vi "MultiplexerSerialInterfaceQueue.vi"() -> ()   [LabVIEW 2016]
uses:
  controls/Enum.ctl
  <vilib>/rvi/errors/niLvFpgaAdjustHostInterfaceError.vi
  <vilib>/regexp/Match Regular Expression.xnode
  <vilib>/rvi/interface/nirviReadWriteControl/nirviReadWriteControl.xnode
  controls/FPGAVIreferenceTypeDef.ctl
  FPGA Bitfiles/qnmController797_usbRIO_controllerFPGAmu.lvbitx
  Course Project/support/Message Queue/Message Queue.lvlib
  NiFpgaLv.dll
panel:
  in  "Clock delay":u32=1
  in  "QuadMultiplier":T1={"Update Multiplexer"=FALSE, "Adress (0-3)"=1, "Resistance"=0} {"Resistance" max=256; "Adress (0-3)" max=32}
  in  "Buffer":T2={"Update Multiplexer"=FALSE, "CH(0-3)"=1, "Output Voltage"=0.0} {"CH(0-3)" max=4}
  in  "VGA":cluster{"Update":bool, "Gain (0-40) (dB)":u32}={"Update"=FALSE, "Gain (0-40) (dB)"=6} {"Gain (0-40) (dB)" max=40}
  in  "Multiplexer":T3={"Update Multiplexer"=FALSE, "Channel #"=2} {"Channel #" max=32}
  in  "Output Enable":bool
  # "Buffer"
  # "VGA"
  # "HMC960LP4E"
  # "DAC8554"
  # "Quad Multiplier"
  # "Multiplexer"
  # "HV5122"
  # "AD5144"
  # "Update the multiplexer"
  # "Offset"
  # "Filter"
  # "Range"
  # "MICROCHIP"
  # "TEXAS INSTRUMENTS"
  # "Serial to Parallel Converter"
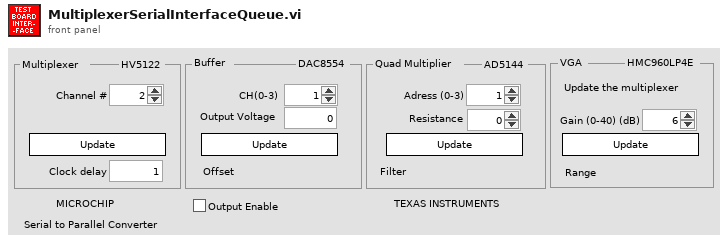
[diagram p1: front panel]
types:
  T1 = cluster{"Update Multiplexer":bool, "Adress (0-3)":u8, "Resistance":u16}
  T2 = cluster{"Update Multiplexer":bool, "CH(0-3)":u8, "Output Voltage":dbl}
  T3 = cluster{"Update Multiplexer":bool, "Channel #":u8}
  T4 = typedef "Message Queue.lvlib/All Message Queues.ctl" = cluster{"IU":refnum<queue>}
  T5 = typedef "Enum.ctl" = enum16{"Init", "Read", "Write"}
  T6 = typedef "FPGAVIreferenceTypeDef.ctl" = refnum<k20>
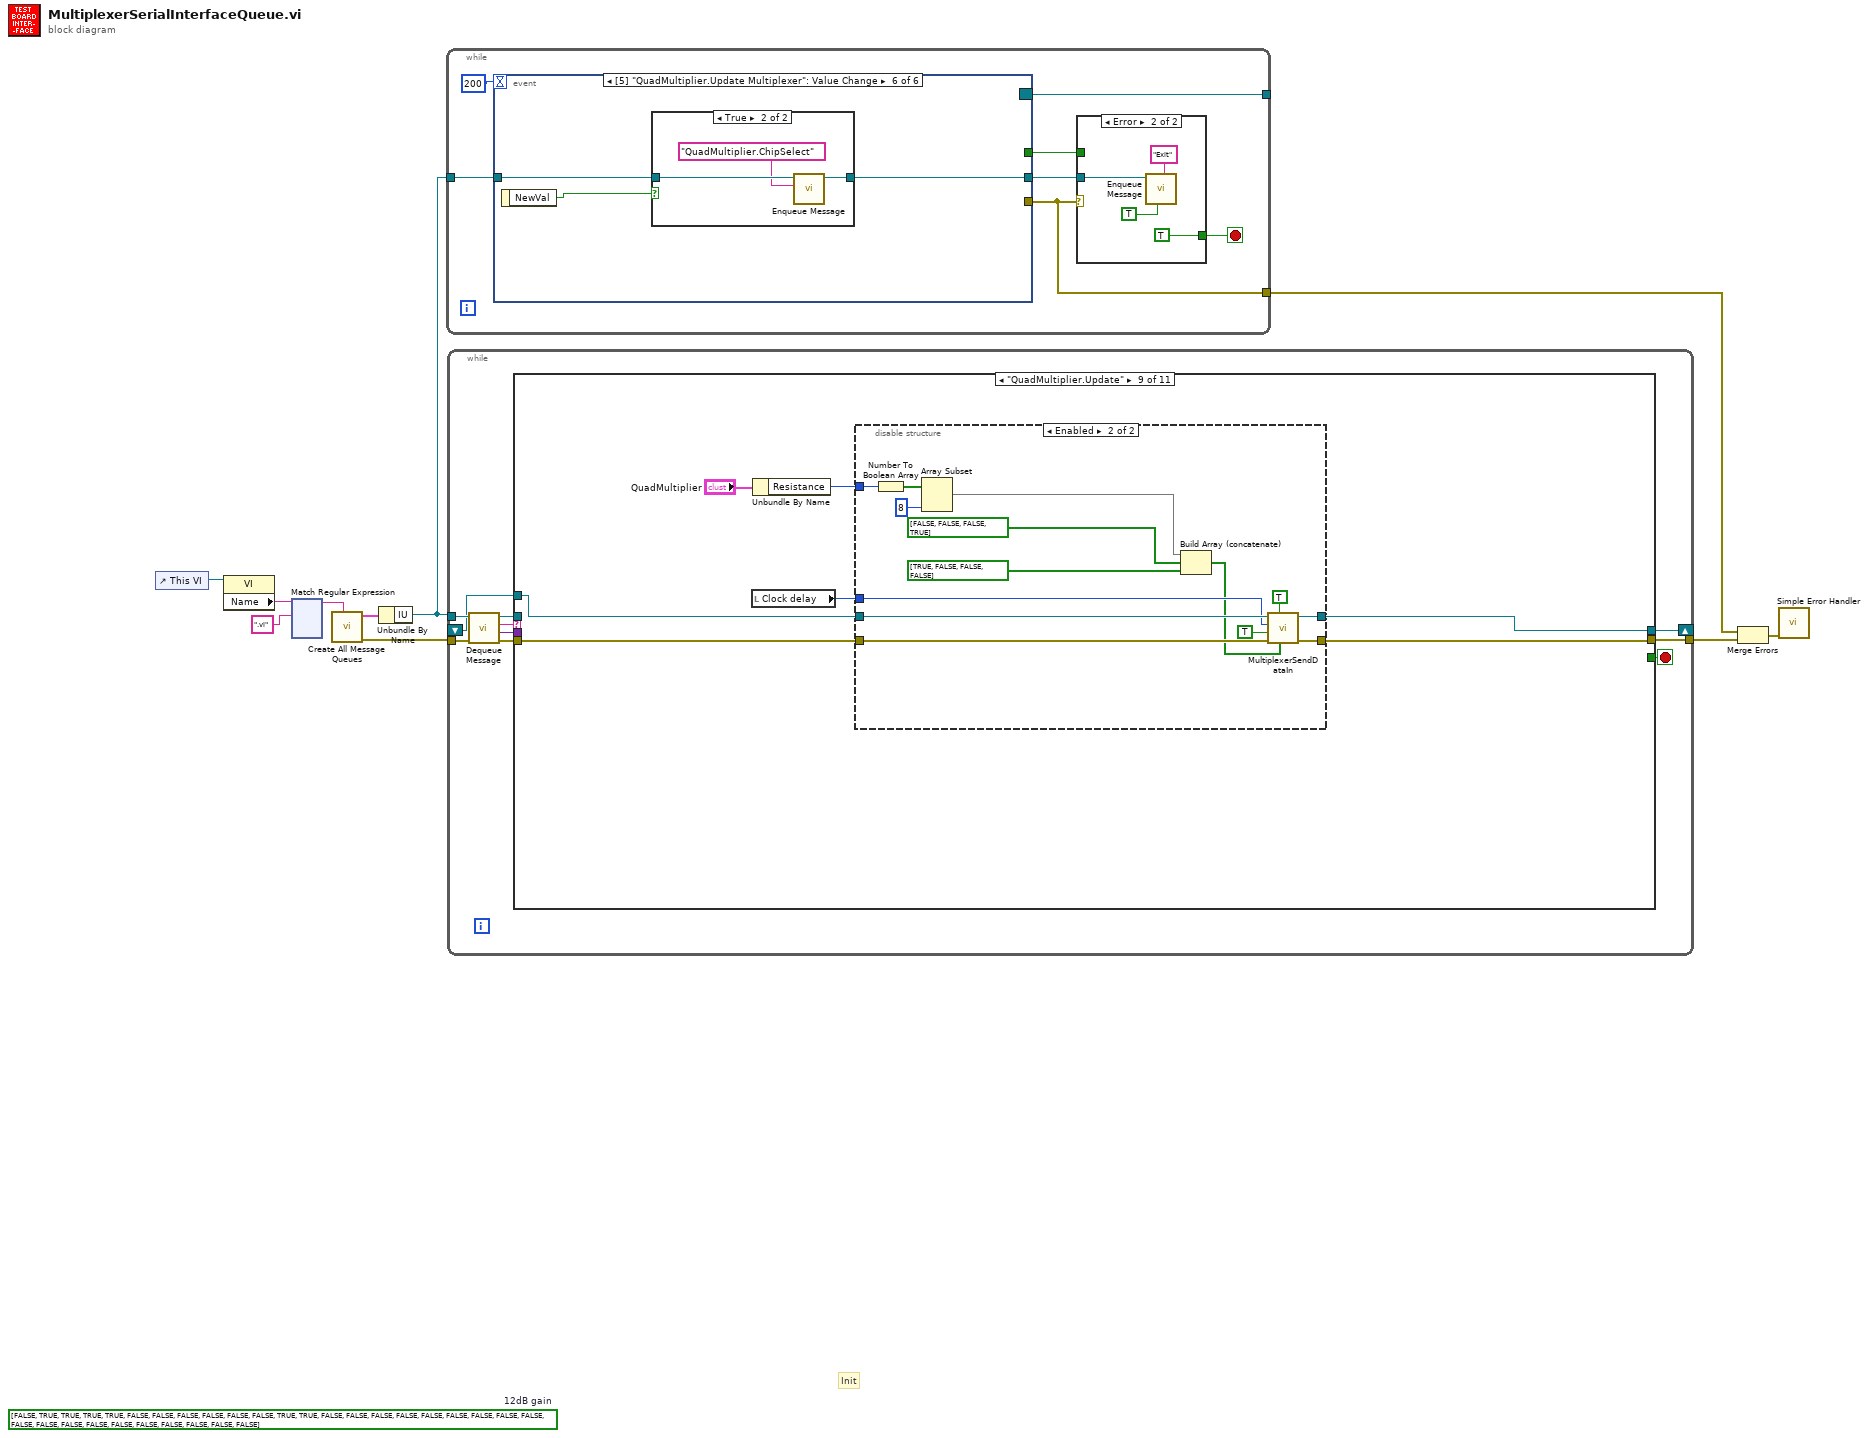
[diagram p0: block diagram]
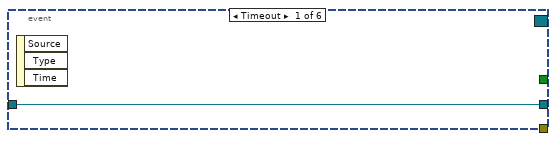
[diagram p3: hidden frame]
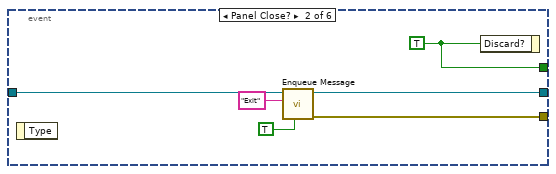
[diagram p4: hidden frame]
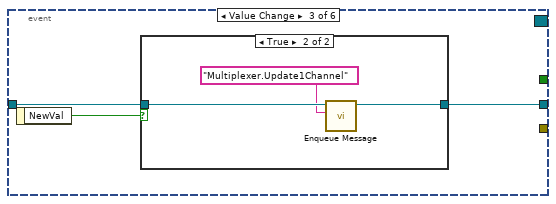
[diagram p5: hidden frame]
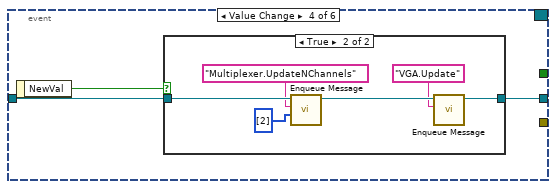
[diagram p7: hidden frame]
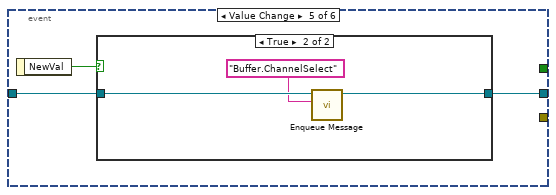
[diagram p9: hidden frame]
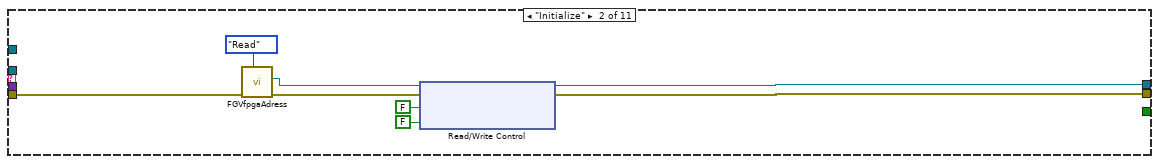
[diagram p13: hidden frame]
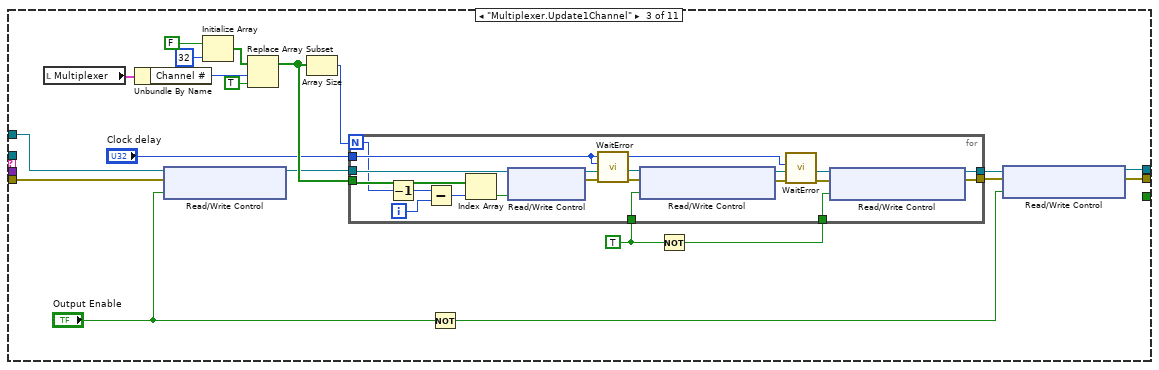
[diagram p14: hidden frame]
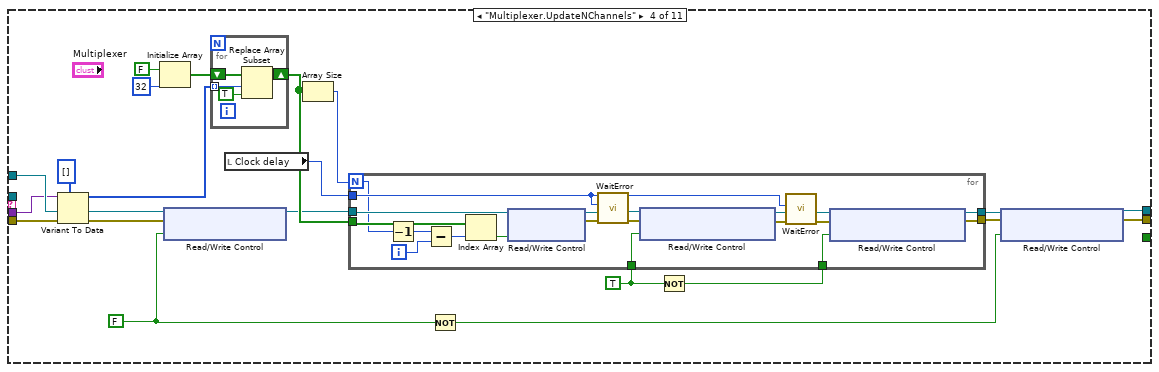
[diagram p15: hidden frame]
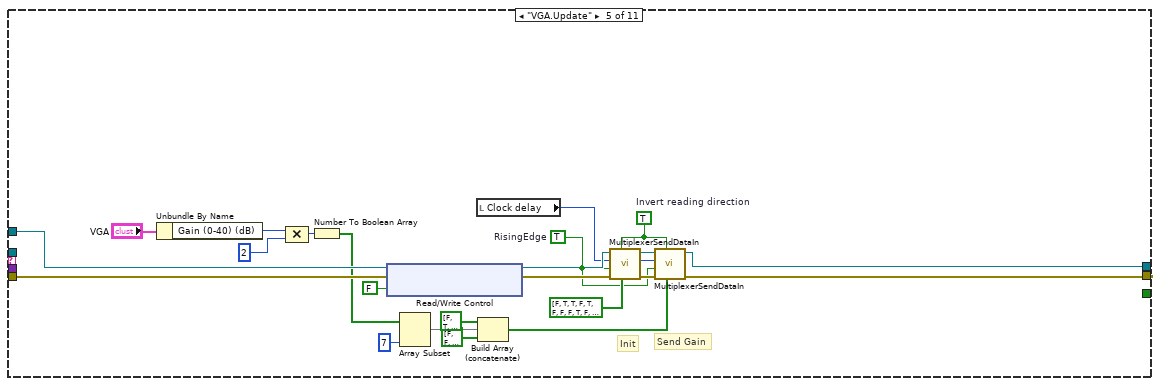
[diagram p16: hidden frame]
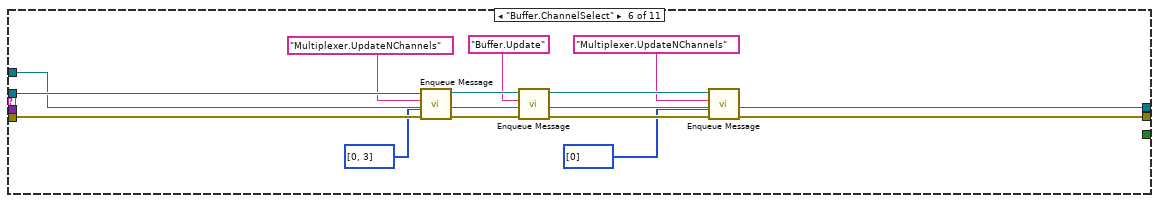
[diagram p17: hidden frame]
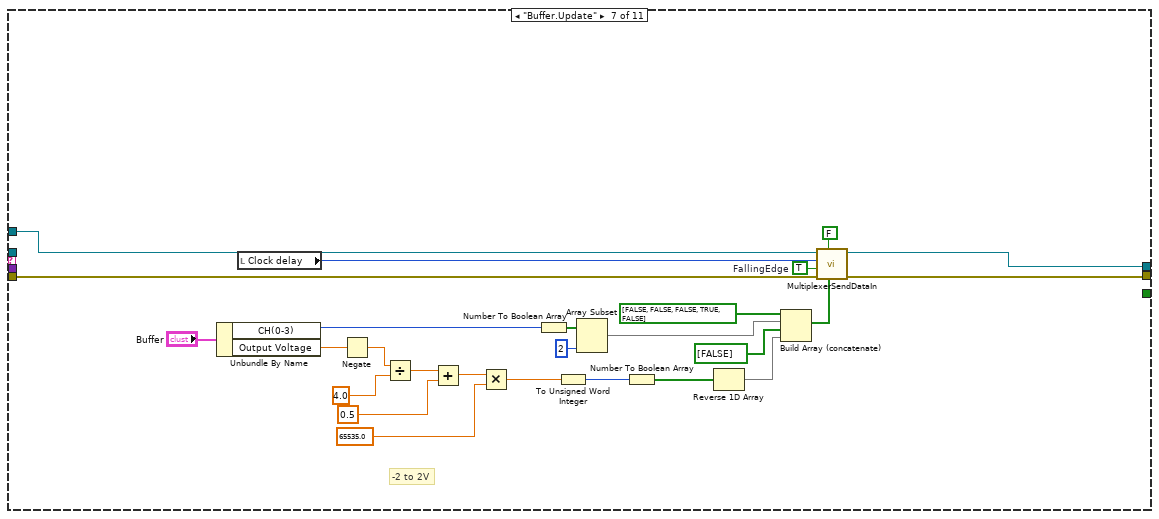
[diagram p18: hidden frame]
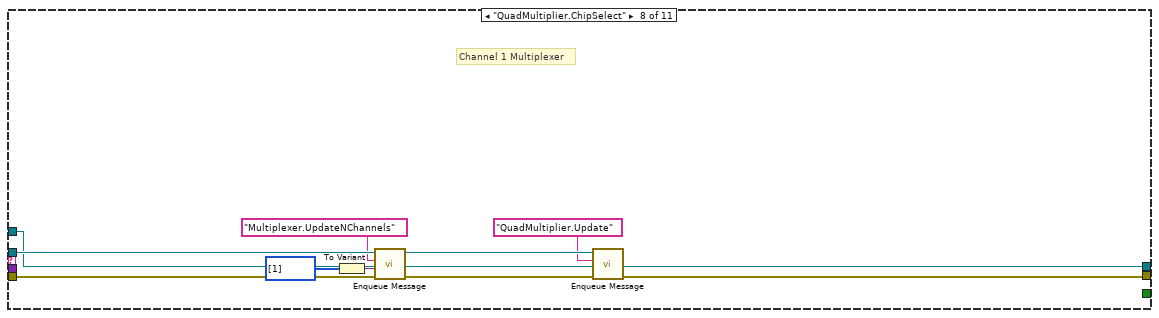
[diagram p19: hidden frame]
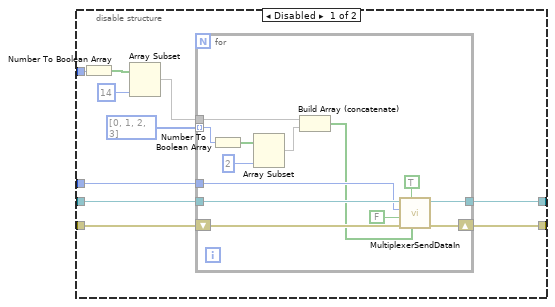
[diagram p20: hidden frame]
diagram:
  (unwired) bool[] [FALSE, TRUE, TRUE, TRUE, TRUE, FALSE, FALSE, FALSE, FALSE, FALSE, FALSE, TRUE, TRUE, FALSE, FALSE, FALSE, FALSE, FALSE, FALSE, FALSE, FALSE, FALSE, FALSE, FALSE, FALSE, FALSE, FALSE, FALSE, FALSE, FALSE, FALSE, FALSE]  # 12dB gain
  # "Init"
  n1 = control-ref of="This VI"() -> (w4:refnum<vi>)
  n2 = property class="VI"(reference=w4) -> ("Name"=w3:string)  [unwired: 1 in, 2 out]
  n3 = xnode "Match Regular Expression"("input string"=w3, "regular expression"=".vi") -> ("before match"=w1:string)  [unwired: 4 in, 4 out]
  n4 = call "Create All Message Queues.vi"("QueueName"=w1) -> ("ErrorOut"=w8:errorcluster, "MessageQueueOut"=w10:T4)  [unwired: 9 in]
  n5 = Unbundle By Name(w10) -> ("IU"=w9:refnum<queue>)
  n6 = while {
    tunnel: w9 -> [w17]
    tunnel: [w13] -> w5
    tunnel: [w12] -> _
    stop <- w15 stop-if-true
    n7 = event shown="[5] \"QuadMultiplier.Update Multiplexer\": Value Change" {
      selector: _ -> [_ _ _ _ _ _]
      dyn-events: [_ _ _ _ _ _] -> w12
      timeout: 200 -> [_ _ _ _ _ _]
      tunnel: [_ w29 _ _ _ _] -> w16
      tunnel: w17 -> [w23 w28 w32 w39 w49 w56]
      tunnel: [_ w27 _ _ _ _] -> w13
      tunnel: [w23 w26 w31 w38 w48 w55] -> w14
      event Timeout {
        n8 = event-data() -> ()  [unwired: 1 in, 3 out]
      }
      event Panel Close? {
        w29 = TRUE ("Rejeter ?")
        n9 = event-data() -> ()  [unwired: 1 in, 1 out]
        n10 = call "Enqueue Message.vi"("Prioritary message"=TRUE ("Message prioritaire ? (F)"), "Message"="Exit", "Queue"=w28) -> ("error out"=w27:errorcluster, "Queue dup."=w26:refnum<queue>)  [unwired: 7 in]
        n11 = event-data ("Event Filter Node")("Discard?"=w29) -> ()  [unwired: 1 in, 1 out]
      }
      event "Multiplexer.Update Multiplexer": Value Change {
        n12 = event-data() -> ("NewVal"=w30:bool)  [unwired: 1 in]
        n13 = case shown="True" w30 {
          tunnel: w32 -> [w33 w36]
          tunnel: [w33 w35] -> w31
          frame False {
          }
          frame True {
            n14 = call "Enqueue Message.vi"("Message"="Multiplexer.Update1Channel", "Queue"=w36) -> ("Queue dup."=w35:refnum<queue>)  [unwired: 8 in, 1 out]
          }
        }
      }
      event "VGA.Update": Value Change {
        n15 = event-data() -> ("NewVal"=w37:bool)  [unwired: 1 in]
        n16 = case shown="True" w37 {
          tunnel: w39 -> [w40 w45]
          tunnel: [w40 w44] -> w38
          frame False {
          }
          frame True {
            n17 = call "Enqueue Message.vi"("Data"=i32[] [2], "Message"="Multiplexer.UpdateNChannels", "Queue"=w45) -> ("Queue dup."=w46:refnum<queue>)  [unwired: 7 in, 1 out]
            n18 = call "Enqueue Message.vi"("Message"="VGA.Update", "Queue"=w46) -> ("Queue dup."=w44:refnum<queue>)  [unwired: 8 in, 1 out]
          }
        }
      }
      event "Buffer.Update Multiplexer": Value Change {
        n19 = event-data() -> ("NewVal"=w47:bool)  [unwired: 1 in]
        n20 = case shown="True" w47 {
          tunnel: w49 -> [w50 w53]
          tunnel: [w50 w51] -> w48
          frame False {
          }
          frame True {
            n21 = call "Enqueue Message.vi"("Message"="Buffer.ChannelSelect", "Queue"=w53) -> ("Queue dup."=w51:refnum<queue>)  [unwired: 8 in, 1 out]
          }
        }
      }
      event "QuadMultiplier.Update Multiplexer": Value Change {
        n22 = event-data() -> ("NewVal"=w54:bool)  [unwired: 1 in]
        n23 = case shown="True" w54 {
          tunnel: w56 -> [w57 w60]
          tunnel: [w57 w59] -> w55
          frame False {
          }
          frame True {
            n24 = call "Enqueue Message.vi"("Message"="QuadMultiplier.ChipSelect", "Queue"=w60) -> ("Queue dup."=w59:refnum<queue>)  [unwired: 8 in, 1 out]
          }
        }
      }
    }
    n25 = case shown="Error" w13 {
      tunnel: [w18 TRUE ("Rejeter ?")] -> w15
      tunnel: w16 -> [w18 _]
      tunnel: w14 -> [_ w21]
      frame No Error {
      }
      frame Error {
        n26 = call "Enqueue Message.vi"("Prioritary message"=TRUE ("Message prioritaire ? (F)"), "Message"="Exit", "Queue"=w21) -> ()  [unwired: 7 in, 2 out]
      }
    }
  }
  n27 = while {
    tunnel: w9 -> [w65]
    tunnel: w8 -> [w69]
    tunnel: [w61] -> w6
    shift-right: [w63] -> _
    shift-left: _ -> [w62]
    stop <- w70 stop-if-true
    n28 = call "Dequeue Message.vi"("entrée d'erreur (pas d'erreur)"=w69, "File d'attente de messages"=w65) -> ("sortie d'erreur"=w68:errorcluster, "Données de message"=w67:variant, "Message"=w64:string, "File d'attente de message dup."=w66:refnum<queue>)  [unwired: 6 in]
    n29 = case "Conditions des messages" shown="\"QuadMultiplier.Update\"" w64 {
      selector: w64 -> [_ _ _ _ _ _ _ _ _ _ w287]
      tunnel: w66 -> [_ _ _ _ _ w197 _ w233 _ w282 _]
      tunnel: w68 -> [w72 w78 w88 w128 w172 w196 w223 w231 w236 w280 _]
      tunnel: [w72 w77 w83 w121 w169 w186 w222 w224 w240 w279 w285] -> w61
      tunnel: [_ _ _ _ _ _ _ _ _ TRUE _] -> w70
      tunnel: w67 -> [_ _ _ w126 _ _ _ _ _ _ _]
      tunnel: [w71 w76 w89 w132 w168 w195 w211 w232 w237 w278 w283] -> w63
      tunnel: w62 -> [w71 _ w91 w134 w173 w195 w212 w232 w238 w278 w283]
      frame "--------- Initialization ---------" {
      }
      frame "Initialize" {
        n30 = call "FGVfpgaAdress.vi"("Enum"=Enum."Read", "error in"=w78) -> ("error out"=w79:errorcluster, "FPGA VI Reference Out"=w80:T6)  [unwired: 4 in, 4 out]
        n31 = xnode "Read/Write Control"("FPGA VI Reference In"=w80, "error in"=w79, "dio.p.multiplexerOE"=FALSE, "dio.p.multiplexerclock"=FALSE) -> ("FPGA VI Reference Out"=w76:T6, "error out"=w77:errorcluster)
      }
      frame "Multiplexer.Update1Channel" {
        w87 = TRUE ("dio.p.multiplexerclock")
        n32 = local read "Multiplexer"() -> (w85:T3)
        n33 = Unbundle By Name(w85) -> ("Channel #"=w99:u8)
        n34 = xnode "Read/Write Control"("FPGA VI Reference In"=w91, "error in"=w88, "dio.p.multiplexerOE"="Output Enable") -> ("FPGA VI Reference Out"=w92:T6)  [unwired: 1 out]
        n35 = Initialize Array(FALSE, 32 ("dimension size")) -> (w98:bool[])
        n36 = Replace Array Subset(array=w98, new element=TRUE ("new element/subarray"), index=w99) -> (w100:bool[])
        n37 = Array Size(array=w100) -> (size(s)=w96:i32)
        n38 = Not(x="Output Enable") -> (.not. x?=w94:bool)
        n39 = Not(x=w87) -> (.not. x?=w86:bool)
        n40 = for {
          N: w96 -> [w108]
          tunnel: "Clock delay" -> [w112]
          tunnel: w92 -> [w111]
          tunnel: w100 -> [w109]
          tunnel: w87 -> [w110]
          tunnel: [w105] -> w90
          tunnel: w86 -> [w104]
          tunnel: [w103] -> w84
          i -> [w107]
          n41 = Decrement(x=w108) -> (x-1=w101:i32)
          n42 = Subtract(x=w101, y=w107) -> (x-y=w106:i32)
          n43 = Index Array(array=w109, index=w106) -> (element=w102:bool)
          n44 = xnode "Read/Write Control"("FPGA VI Reference In"=w111, "dio.i.dataIn"=w102) -> ("FPGA VI Reference Out"=w113:T6, "error out"=w118:errorcluster)  [unwired: 1 in]
          n45 = call "WaitError.vi"("error in (no error)"=w118, "milliseconds to wait"=w112) -> ("error out"=w117:errorcluster)  [unwired: 9 in]
          n46 = xnode "Read/Write Control"("FPGA VI Reference In"=w113, "error in"=w117, "dio.p.multiplexerclock"=w110) -> ("FPGA VI Reference Out"=w114:T6, "error out"=w116:errorcluster)
          n47 = call "WaitError.vi"("error in (no error)"=w116, "milliseconds to wait"=w112) -> ("error out"=w115:errorcluster)  [unwired: 9 in]
          n48 = xnode "Read/Write Control"("FPGA VI Reference In"=w114, "error in"=w115, "dio.p.multiplexerclock"=w104) -> ("FPGA VI Reference Out"=w105:T6, "error out"=w103:errorcluster)
        }
        n49 = xnode "Read/Write Control"("FPGA VI Reference In"=w90, "error in"=w84, "dio.p.multiplexerOE"=w94) -> ("FPGA VI Reference Out"=w89:T6, "error out"=w83:errorcluster)
      }
      frame "Multiplexer.UpdateNChannels" {
        w129 = FALSE ("x")
        w131 = TRUE ("dio.p.multiplexerclock")
        n50 = Variant To Data(error in=w128, type=i32[] [], Variant=w126) -> (data=w123:i32[], error out=w127:errorcluster)
        n51 = Initialize Array(FALSE, 32 ("dimension size")) -> (w124:bool[])
        n52 = xnode "Read/Write Control"("FPGA VI Reference In"=w134, "error in"=w127, "dio.p.multiplexerOE"=w129) -> ("FPGA VI Reference Out"=w135:T6)  [unwired: 1 out]
        n53 = for {
          shift-right: [w143] -> w139
          shift-left: w124 -> [w141]
          tunnel: w123 -> [w140] mode=indexing
          n54 = Replace Array Subset(array=w141, new element=TRUE ("new element/subarray"), index=w140) -> (w143:bool[])
        }
        n55 = local read "Clock delay"() -> (w120:u32)
        n56 = Array Size(array=w139) -> (size(s)=w137:i32)
        n57 = Not(x=w129) -> (.not. x?=w136:bool)
        n58 = Not(x=w131) -> (.not. x?=w130:bool)
        n59 = for {
          N: w137 -> [w151]
          tunnel: w120 -> [w155]
          tunnel: w135 -> [w154]
          tunnel: w139 -> [w152]
          tunnel: w131 -> [w153]
          tunnel: [w148] -> w133
          tunnel: w130 -> [w147]
          tunnel: [w146] -> w122
          i -> [w150]
          n60 = Decrement(x=w151) -> (x-1=w144:i32)
          n61 = Subtract(x=w144, y=w150) -> (x-y=w149:i32)
          n62 = Index Array(array=w152, index=w149) -> (element=w145:bool)
          n63 = xnode "Read/Write Control"("FPGA VI Reference In"=w154, "dio.i.dataIn"=w145) -> ("FPGA VI Reference Out"=w156:T6, "error out"=w161:errorcluster)  [unwired: 1 in]
          n64 = call "WaitError.vi"("error in (no error)"=w161, "milliseconds to wait"=w155) -> ("error out"=w160:errorcluster)  [unwired: 9 in]
          n65 = xnode "Read/Write Control"("FPGA VI Reference In"=w156, "error in"=w160, "dio.p.multiplexerclock"=w153) -> ("FPGA VI Reference Out"=w157:T6, "error out"=w159:errorcluster)
          n66 = call "WaitError.vi"("error in (no error)"=w159, "milliseconds to wait"=w155) -> ("error out"=w158:errorcluster)  [unwired: 9 in]
          n67 = xnode "Read/Write Control"("FPGA VI Reference In"=w157, "error in"=w158, "dio.p.multiplexerclock"=w147) -> ("FPGA VI Reference Out"=w148:T6, "error out"=w146:errorcluster)
        }
        n68 = xnode "Read/Write Control"("FPGA VI Reference In"=w133, "error in"=w122, "dio.p.multiplexerOE"=w136) -> ("FPGA VI Reference Out"=w132:T6, "error out"=w121:errorcluster)
      }
      frame "VGA.Update" {
        w163 = TRUE  # RisingEdge
        w166 = TRUE  # Invert reading direction
        # "Send Gain"
        # "Init"
        n69 = Unbundle By Name("VGA") -> ("Gain (0-40) (dB)"=w179:u32)
        n70 = Compound Arithmetic op=MULTIPLY(w179, u32 2 ("value")) -> (w180:u32)
        n71 = Number To Boolean Array(number=w180) -> (Boolean array=w167:bool[])
        n72 = xnode "Read/Write Control"("FPGA VI Reference In"=w173, "error in"=w172, "dio.p.multiplexerclock"=FALSE) -> ("FPGA VI Reference Out"=w175:T6, "error out"=w177:errorcluster)
        n73 = Array Subset(array=w167, length=7) -> (w182:bool[])  [unwired: 1 in]
        n74 = local read "Clock delay"() -> (w162:u32)
        n75 = Build Array (concatenate)(bool[] [FALSE, TRUE, TRUE, TRUE, TRUE, FALSE, FALSE, FALSE], w182, bool[] [FALSE, FALSE, FALSE, FALSE, FALSE, FALSE, FALSE, FALSE, FALSE, FALSE, FALSE, FALSE, FALSE, FALSE, FALSE, FALSE, FALSE]) -> (w170:bool[])
        n76 = call "MultiplexerSendDataIn.vi"("DataIn"=bool[] [FALSE, TRUE, TRUE, FALSE, TRUE, FALSE, FALSE, FALSE, TRUE, FALSE, FALSE, TRUE, TRUE, TRUE, FALSE, FALSE, FALSE, FALSE, FALSE, FALSE, FALSE, FALSE, FALSE, FALSE, FALSE, FALSE, FALSE, FALSE, FALSE, FALSE, FALSE, FALSE] ("output array"), "Invert"=w166, "error in"=w177, "RisingEdge"=w163, "Clock delay"=w162, "Refnum in"=w175) -> ("error out"=w165:errorcluster, "Refnum out"=w164:T6)  [unwired: 4 in]
        n77 = call "MultiplexerSendDataIn.vi"("DataIn"=w170, "Invert"=w166, "error in"=w165, "RisingEdge"=w163, "Clock delay"=w162, "Refnum in"=w164) -> ("error out"=w169:errorcluster, "Refnum out"=w168:T6)  [unwired: 4 in]
      }
      frame "Buffer.ChannelSelect" {
        n78 = call "Enqueue Message.vi"("error in"=w196, "Data"=i32[] [0, 3], "Message"="Multiplexer.UpdateNChannels", "Queue"=w197) -> ("error out"=w190:errorcluster, "Queue dup."=w194:refnum<queue>)  [unwired: 6 in]
        n79 = call "Enqueue Message.vi"("error in"=w190, "Message"="Buffer.Update", "Queue"=w194) -> ("error out"=w187:errorcluster, "Queue dup."=w189:refnum<queue>)  [unwired: 7 in]
        n80 = call "Enqueue Message.vi"("error in"=w187, "Data"=i32[] [0], "Message"="Multiplexer.UpdateNChannels", "Queue"=w189) -> ("error out"=w186:errorcluster)  [unwired: 6 in, 1 out]
      }
      frame "Buffer.Update" {
        w209 = TRUE  # FallingEdge
        # "-2 to 2V"
        n81 = Unbundle By Name("Buffer") -> ("CH(0-3)"=w219:u8, "Output Voltage"=w201:dbl)
        n82 = local read "Clock delay"() -> (w202:u32)
        n83 = Negate(x=w201) -> (-x=w198:dbl)
        n84 = Divide(x=w198, y=4.0) -> (x/y=w206:dbl)
        n85 = Add(x=w206, y=0.5) -> (x+y=w204:dbl)
        n86 = Multiply(x=w204, y=65535.0) -> (x*y=w200:dbl)
        n87 = Number To Boolean Array(number=w219) -> (Boolean array=w218:bool[])
        n88 = To Unsigned Word Integer(number=w200) -> (unsigned 16bit integer=w199:u16)
        n89 = Array Subset(array=w218, length=2) -> (w216:bool[])  [unwired: 1 in]
        n90 = Number To Boolean Array(number=w199) -> (Boolean array=w214:bool[])
        n91 = Reverse 1D Array(array=w214) -> (reversed array=w208:bool[])
        n92 = Build Array (concatenate)(bool[] [FALSE, FALSE, FALSE, TRUE, FALSE], w216, bool[] [FALSE] ("array"), w208) -> (w213:bool[])
        n93 = call "MultiplexerSendDataIn.vi"("DataIn"=w213, "Invert"=FALSE, "error in"=w223, "RisingEdge"=w209, "Clock delay"=w202, "Refnum in"=w212) -> ("error out"=w222:errorcluster, "Refnum out"=w211:T6)  [unwired: 4 in]
      }
      frame "QuadMultiplier.ChipSelect" {
        # "Channel 1 Multiplexer"
        n94 = To Variant(anything=i32[] [1]) -> (Variant=w229:variant)
        n95 = call "Enqueue Message.vi"("error in"=w231, "Data"=w229, "Message"="Multiplexer.UpdateNChannels" ("QueueName"), "Queue"=w233) -> ("error out"=w225:errorcluster, "Queue dup."=w227:refnum<queue>)  [unwired: 6 in]
        n96 = call "Enqueue Message.vi"("error in"=w225, "Message"="QuadMultiplier.Update", "Queue"=w227) -> ("error out"=w224:errorcluster)  [unwired: 7 in, 1 out]
      }
      frame "QuadMultiplier.Update" {
        n97 = local read "Clock delay"() -> (w234:u32)
        n98 = Unbundle By Name("QuadMultiplier") -> ("Resistance"=w235:u16)
        n99 = disable-structure shown="Enabled" {
          disable-tunnel: [w250 w272] -> w240
          disable-tunnel: w238 -> [w249 w274]
          disable-tunnel: [w248 w273] -> w237
          disable-tunnel: w236 -> [w247 w271]
          disable-tunnel: w235 -> [w246 w275]
          disable-tunnel: w234 -> [w241 w270]
          frame Disabled {
            n100 = Number To Boolean Array(number=w246) -> (Boolean array=w244:bool[])
            n101 = Array Subset(array=w244, length=14 ("index")) -> (w245:bool[])  [unwired: 1 in]
            n102 = for {
              tunnel: w249 -> [w260]
              tunnel: [w259] -> w248
              tunnel: w241 -> [w258]
              tunnel: i32[] [0, 1, 2, 3] -> [w254] mode=indexing
              shift-right: [w262] -> w250
              shift-left: w247 -> [w263]
              tunnel: w245 -> [w255]
              n103 = Number To Boolean Array(number=w254) -> (Boolean array=w253:bool[])
              n104 = Array Subset(array=w253, length=2 ("index")) -> (w252:bool[])  [unwired: 1 in]
              n105 = Build Array (concatenate)(w255, w252) -> (w256:bool[])
              n106 = call "MultiplexerSendDataIn.vi"("DataIn"=w256, "Invert"=TRUE, "error in"=w263, "RisingEdge"=FALSE, "Clock delay"=w258, "Refnum in"=w260) -> ("error out"=w262:errorcluster, "Refnum out"=w259:T6)  [unwired: 4 in]
            }
          }
          frame Enabled {
            n107 = Number To Boolean Array(number=w275) -> (Boolean array=w277:bool[])
            n108 = Array Subset(array=w277, length=8 ("index")) -> (w268:bool[])  [unwired: 1 in]
            n109 = Build Array (concatenate)(w268, bool[] [FALSE, FALSE, FALSE, TRUE] ("array"), bool[] [TRUE, FALSE, FALSE, FALSE] ("array")) -> (w265:bool[])
            n110 = call "MultiplexerSendDataIn.vi"("DataIn"=w265, "Invert"=TRUE, "error in"=w271, "RisingEdge"=TRUE, "Clock delay"=w270, "Refnum in"=w274) -> ("error out"=w272:errorcluster, "Refnum out"=w273:T6)  [unwired: 4 in]
          }
        }
      }
      frame "Exit" {
        n111 = Release Queue(queue=w282, error in (no error)=w280) -> (error out=w279:errorcluster)  [unwired: 1 in, 2 out]
      }
      frame Default {
        n112 = Format Into String(format string="The message\"%s\" received in the gestion loop is not valid" ("Texte de message d'erreur inconnu"), w287) -> (resulting string=w284:string)  [unwired: 2 in, 1 out]
        n113 = call <vilib>:"Error Cluster From Error Code.vi"("error message (\"\")"=w284, "error code (0)"=1 ("code d'erreur (0)")) -> ("error out"=w285:errorcluster)  [unwired: 7 in]
      }
    }
  }
  n114 = Merge Errors(w5, w6) -> (w7:errorcluster)
  n115 = call <vilib>:"Simple Error Handler.vi"("error in (no error)"=w7) -> ()  [unwired: 4 in, 5 out]
